vi "Initialize Click Zones Array.vi"(11 "size":i32) -> (3 "array":T2)   [LabVIEW 2017, in "NI_Robotics_Configure Steering Frame.lvlib"]
uses:
  <vilib>/robotics/Dialog/Configure Steering Frame/NI_Robotics_Configure Steering Frame.lvlib
  <vilib>/robotics/Dialog/Configure Steering Frame/Click Zone.ctl
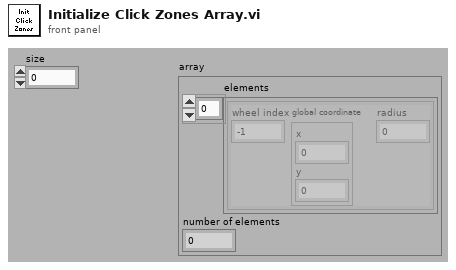
[diagram p1: front panel]
types:
  T1 = typedef "NI_Robotics_Configure Steering Frame.lvlib/Click Zone.ctl" = cluster{"wheel index":i32, "global coordinate":cluster{"x":dbl, "y":dbl}, "radius":dbl}
  T2 = cluster{"elements":T1[], "number of elements":i32}
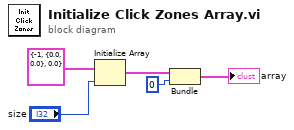
[diagram p0: block diagram]
diagram:
  n1 = Initialize Array(T1 {"wheel index"=-1, "global coordinate"={"x"=0.0, "y"=0.0}, "radius"=0.0} ("click zone"), "size") -> (w2:T1[])
  n2 = Bundle(w2, "size"=0) -> (→"array":cluster{T1[], "size":i32})  [unwired: 1 in]
